vi "SPI Simulation Plotter.vi"(8 "Other Signals":bool[](array[boolean]), 9 "Engine Clock Rate (MHz)":i32=120000000 format="%.0p", 10 "SPI Signals":T2, 11 "SPI PHY Settings":T3={"Divide Value"=10, "Transfer Length (bits)"=24, "CS Asserted Polarity"=FALSE, "Clock Polarity (CPOL)"=FALSE, "Clock Phase (CPHA)"=FALSE, "Lengthen MISO Setup"=FALSE, "Direction Change Bit"=0, "MOSI Starts as Output"=FALSE, "Tristatable MOSI"=FALSE}) -> (2 "Timing Characteristics":T1 {"tCP (ns)" format="%#_4g"; "tCSS (ns)" format="%#_4g"; "tCSH (ns)" format="%#_4g"; "tCSW (ns)" format="%#_4g"; "Actual Sample Rate (Hz)" format="%_4p"; "SCLK Frequency (Hz)" format="%#.2p"}, 3 "Digital Data":digitalwaveform(graph), 5 "Chart Size":i32)   [LabVIEW 2015]
uses:
  Controls/Digital Data.ctl
  Controls/Timing Characteristics.ctl
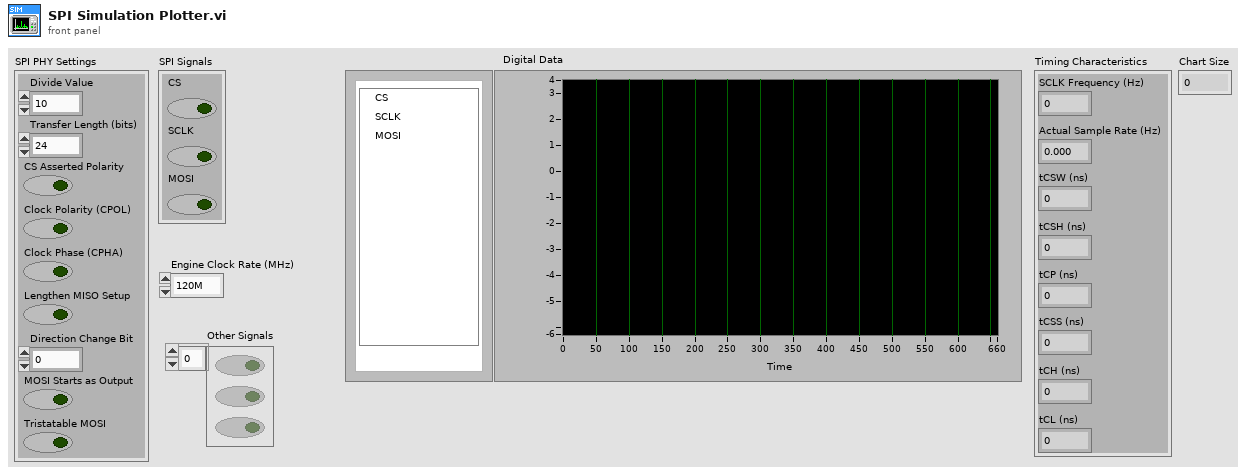
[diagram p1: front panel]
types:
  T1 = typedef "Timing Characteristics.ctl" = cluster{"SCLK Frequency (Hz)":dbl, "Actual Sample Rate (Hz)":dbl, "tCSW (ns)":dbl, "tCSH (ns)":dbl, "tCSS (ns)":dbl, "tCP (ns)":dbl, "tCH (ns)":dbl, "tCL (ns)":dbl}
  T2 = typedef "Digital Data.ctl" = cluster{"CS":bool, "SCLK":bool, "MOSI":bool}
  T3 = cluster{"Divide Value":u8, "Transfer Length (bits)":u8, "CS Asserted Polarity":bool, "Clock Polarity (CPOL)":bool, "Clock Phase (CPHA)":bool, "Lengthen MISO Setup":bool, "Direction Change Bit":u8, "MOSI Starts as Output":bool, "Tristatable MOSI":bool}
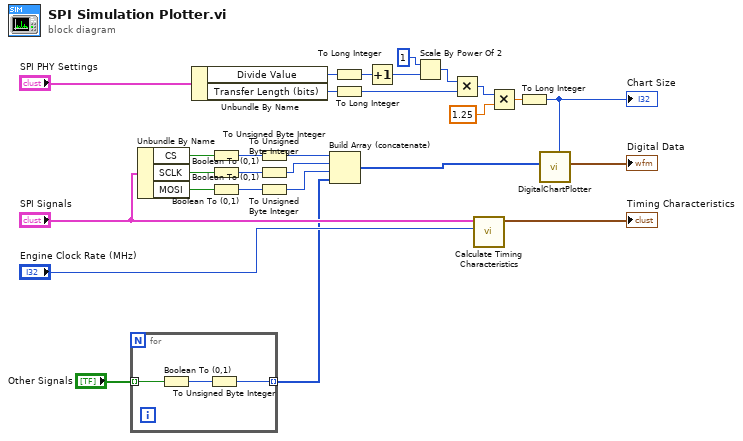
[diagram p0: block diagram]
diagram:
  n1 = for {
    tunnel: "Other Signals" -> [w30] mode=indexing
    tunnel: [w29] -> w1 mode=indexing
    n2 = Boolean To (0,1)(Boolean=w30) -> (0, 1=w31:i16)
    n3 = To Unsigned Byte Integer(number=w31) -> (unsigned 8bit integer=w29:u8)
  }
  n4 = Unbundle By Name("SPI Signals") -> ("CS"=w21:bool, "SCLK"=w20:bool, "MOSI"=w19:bool)
  n5 = Unbundle By Name("SPI PHY Settings") -> ("Divide Value"=w6:u8, "Transfer Length (bits)"=w7:u8)
  n6 = Boolean To (0,1)(Boolean=w21) -> (0, 1=w17:i16)
  n7 = Boolean To (0,1)(Boolean=w20) -> (0, 1=w16:i16)
  n8 = Boolean To (0,1)(Boolean=w19) -> (0, 1=w15:i16)
  n9 = To Unsigned Byte Integer(number=w17) -> (unsigned 8bit integer=w14:u8)
  n10 = To Unsigned Byte Integer(number=w16) -> (unsigned 8bit integer=w13:u8)
  n11 = To Unsigned Byte Integer(number=w15) -> (unsigned 8bit integer=w12:u8)
  n12 = Build Array (concatenate)(w14, w13, w12, w1) -> (w18:u8[])
  n13 = To Long Integer(number=w6) -> (32bit integer=w5:i32)
  n14 = To Long Integer(number=w7) -> (32bit integer=w4:i32)
  n15 = Increment(x=w5) -> (x+1=w25:i32)
  n16 = Scale By Power Of 2(n=i16 1, x=w25) -> (x*2^n=w24:i32)
  n17 = Multiply(x=w24, y=w4) -> (x*y=w27:i32)
  n18 = call "Calculate Timing Characteristics.vi"("Engine Clock Rate (MHz)"="Engine Clock Rate (MHz)", "SPI Signals"="SPI Signals") -> ("Timing Characteristics"=→"Timing Characteristics":T1)  [unwired: 9 in]
  n19 = Multiply(x=w27, y=1.25 ("History Scale")) -> (x*y=w23:dbl)
  n20 = To Long Integer(number=w23) -> (32bit integer=w10:i32)
  "Chart Size" <- w10
  n21 = call "DigitalChartPlotter.vi"("History Size"=w10, "Input"=w18) -> ("Digital Data"=→"Digital Data":digitalwaveform)  [unwired: 9 in]
